vi "16 Relay Ethernet.vi"() -> ()   [LabVIEW 2017]
panel:
  in  "tableau d'octets non signés 2":u8[](array[numeric])=[12, 41, 171, 124, 0, 1, 108, 113, 217, 31, 198, 65, 8, 0, 69, 0, 0, 48, 111, 152, 64, 0, 128, 6, 7, 193, 192, 168, 1, 26, 192, 168, 1, 4, 214, 0, 11, 184, 114, 220, 20, 37, 193, 253, 187, 189, 80, 24, 250, 216, 223, 153, 0, 0, 88, 1, 19, 0, 0, 0, 0, 108] format="%x"
  out "octets écrits":i32
  out "tableau d'octets non signés":u8[](array[numeric])
  # "16 relay communication network protocol\nagreement?TCP/IP\nIP: 192.168.1.4\nport number?3000 \ncode for the control of relay:\n1channel on? 58 01 12 00 00 00 01 6C     1 channel off? 58 01 11 00 00 00 01 6B\n2channel on? 58 01 12 00 00 00 02 6D     2channel off? 58 01 11 00 00 00 02 6C\n3channel on? 58 01 12 00 00 00 03 6E     3channel off? 58 01 11 00 00 00 03 6D\n4channel on? 58 01 12 00 00 00 04 6F     4channel off? 58 01 11 00 00 00 04 6E\n5channel on? 58 01 12 00 00 00 05 70     5channel off? 58 01 11 00 00 00 05 6F\n6channel on? 58 01 12 00 00 00 06 71     6channel off? 58 01 11 00 00 00 06 70\n7channel on? 58 01 12 00 00 00 07 72     7channel off? 58 01 11 00 00 00 07 71\n8channel on? 58 01 12 00 00 00 08 73     8channel off? 58 01 11 00 00 00 08 72\n9channel on? 58 01 12 00 00 00 09 74     9channel off? 58 01 11 00 00 00 09 73\n10channel on? 58 01 12 00 00 00 0A 75    10channel off? 58 01 11 00 00 00 0A 74\n11channel on? 58 01 12 00 00 00 0B 76    11channel off? 58 01 11 00 00 00 0B 75\n12channel on? 58 01 12 00 00 00 0C 77    12channel off? 58 01 11 00 00 00 0C 76\n13channel on? 58 01 12 00 00 00 0D 78    13channel off? 58 01 11 00 00 00 0D 77\n14channel on? 58 01 12 00 00 00 0E 79    14channel off? 58 01 11 00 00 00 0E 78\n15channel on? 58 01 12 00 00 00 0F 7A    15channel off? 58 01 11 00 00 00 0F 79\n16channel on? 58 01 12 00 00 00 10 7B    16channel off? 58 01 11 00 00 00 10 7A\n\n58 01 13 00 00 ff ff 6a                                                                       58 01 13 00 00 00 00 6c\n1-16channel on? 58 01 13 00 00 FF FF 77    1-16channel off?58 01 13 00 00 00 00 7B\n\nQuery the current 16 relay state?58 01 10 00 00 00 00 69\nThe next crew to respond to relay status?   28 01 00 00 00 XX XX HH   (XX XX 16 bit, each bit represents one relay state, \"1\" indicates on, \"0\" indicates OFF; HH is the sum of all previous data together)\n0000   0c 29 ab 7c 00 01 04 92 26 da 58 ff 08 00 45 00   .).|....&.X...E.\n0010   00 30 54 af 40 00 80 06 22 b2 c0 a8 01 12 c0 a8   .0T.@...\".......\n0020   01 04 8c f1 0b b8 80 16 0d 85 e7 86 8e a2 50 18   ..............P.\n0030   fa d8 29 ab 00 00 58 01 13 00 00 ff ff 6a         ..)...X......j\n0000   0c 29 ab 7c 00 01 04 92 26 da 58 ff 08 00 45 00   .).|....&.X...E.\n0010   00 30 54 b1 40 00 80 06 22 b0 c0 a8 01 12 c0 a8   .0T.@...\".......\n0020   01 04 8c f1 0b b8 80 16 0d 8d e7 86 8e aa 50 18   ..............P.\n0030   fa d0 29 a1 00 00 58 01 13 00 00 00 00 6c         ..)...X......l"
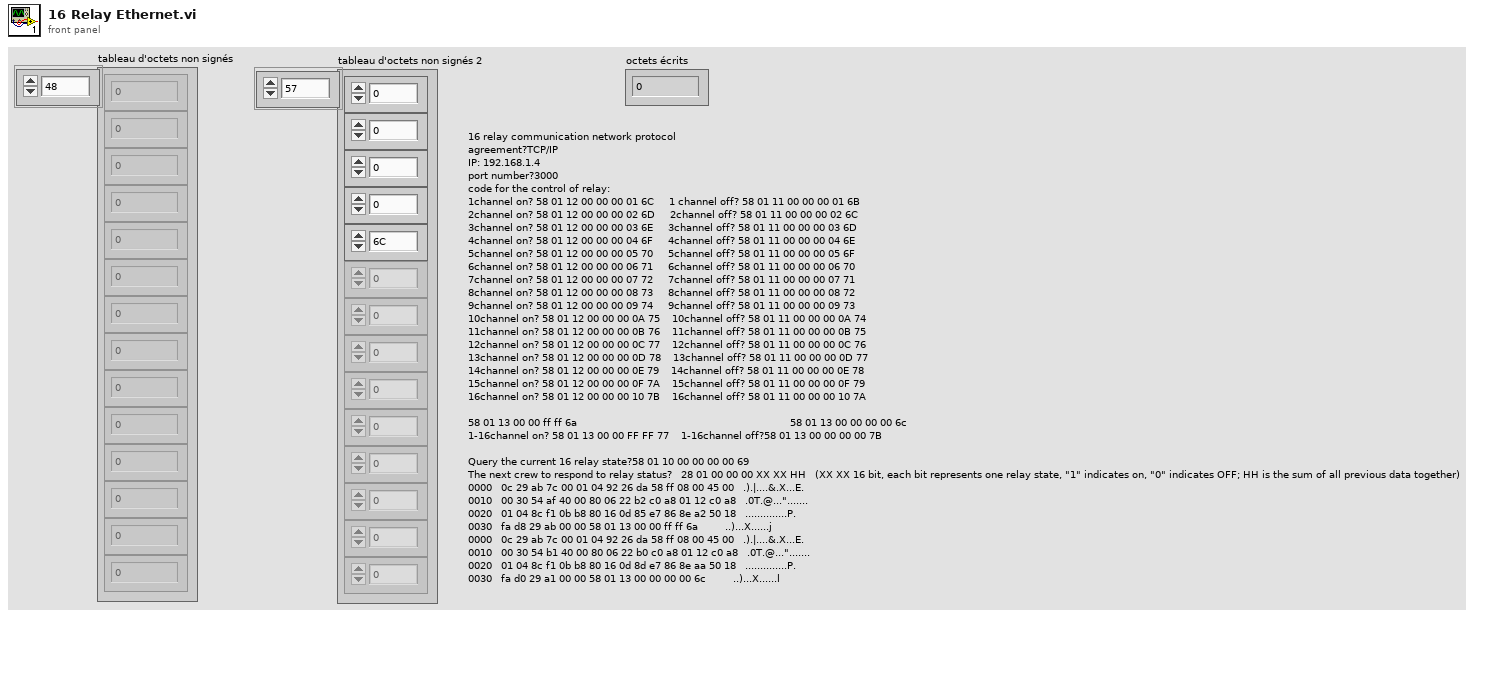
[diagram p1: front panel]
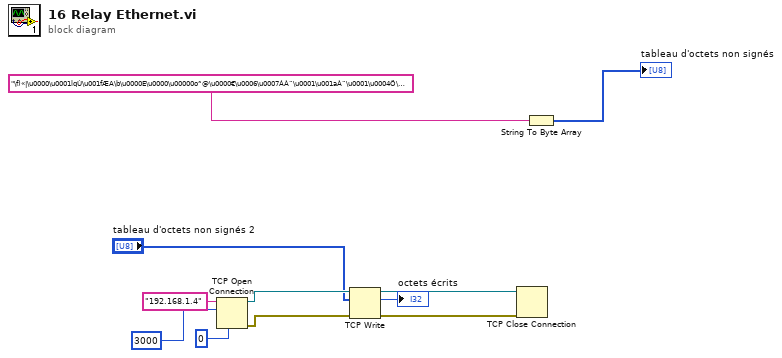
[diagram p0: block diagram]
diagram:
  n1 = TCP Open Connection(address="192.168.1.4" ("adresse"), remote port or service name=u16 3000 ("port distant ou nom du service"), local port=u16 0 ("port local (0)")) -> (connection ID=w11:refnum<k5>, error out=w5:errorcluster)  [unwired: 2 in]
  n2 = TCP Write(connection ID=w11, data in="tableau d'octets non signés 2", error in (no error)=w5) -> (connection ID out=w10:refnum<k5>, bytes written=→"octets écrits":i32, error out=w4:errorcluster)  [unwired: 1 in]
  n3 = TCP Close Connection(connection ID=w10, error in (no error)=w4) -> ()  [unwired: 1 in, 2 out]
  n4 = String To Byte Array(string="\f)«|\u0000\u0001lqÙ\u001fÆA\b\u0000E\u0000\u00000o˜@\u0000€\u0006\u0007ÁÀ¨\u0001\u001aÀ¨\u0001\u0004Ö\u0000\u000b¸rÜ\u0014%Áý»½P\u0018úØß™\u0000\u0000X\u0001\u0012\u0000\u0000\u0000\u0001l" ("données en entrée")) -> (unsigned byte array=→"tableau d'octets non signés":u8[])
